vi "test20-LosslessRegisterStateMultipleTimes.vi"(8 "error in (no error)":errorcluster, 11 "TestCase in":refnum<class "testcase-CSMBroadcast.lvclass">) -> (0 "error out":errorcluster, 3 "TestCase out":refnum<class "testcase-CSMBroadcast.lvclass">)   [LabVIEW 2017, in "testcase-CSMBroadcast.lvclass"]
uses:
  testcase-CSMBroadcast.lvclass
  bc269a46-fbd8-4fbd-ac76-06990d02385a.vi
  8d37a2f4-20d8-4102-818c-5a8acec6f80e.vi
  src/user.lib/_NEVSTOP/Communicable State Machine(CSM)/AdvanceAPI/CSM - Get Module Attribute.vi
  <vilib>/addons/_JKI Toolkits/VI Tester/TestCase.llb/TestCase.lvclass
  src/user.lib/_NEVSTOP/Communicable State Machine(CSM)/Communicable State Machine.lvlib
  C:/Program Files (x86)/National Instruments/LabVIEW 2017/vi.lib/addons/_JKI Toolkits/VI Tester/TestCase.llb/TestCase.lvclass
panel:
  out "error out 2":errorcluster
  out "LoopCount":i32
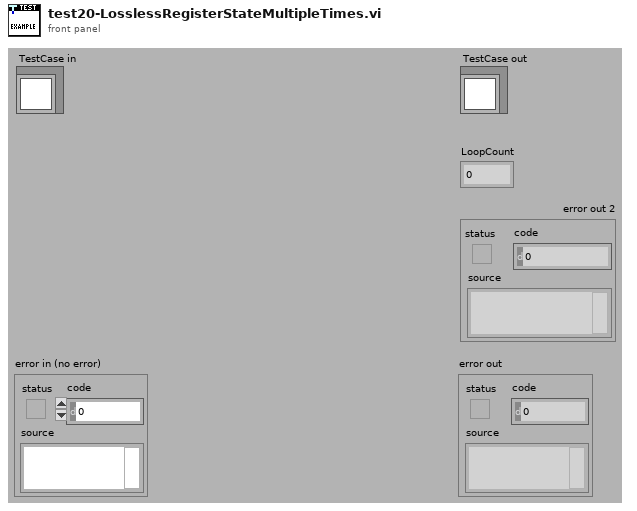
[diagram p1: front panel]
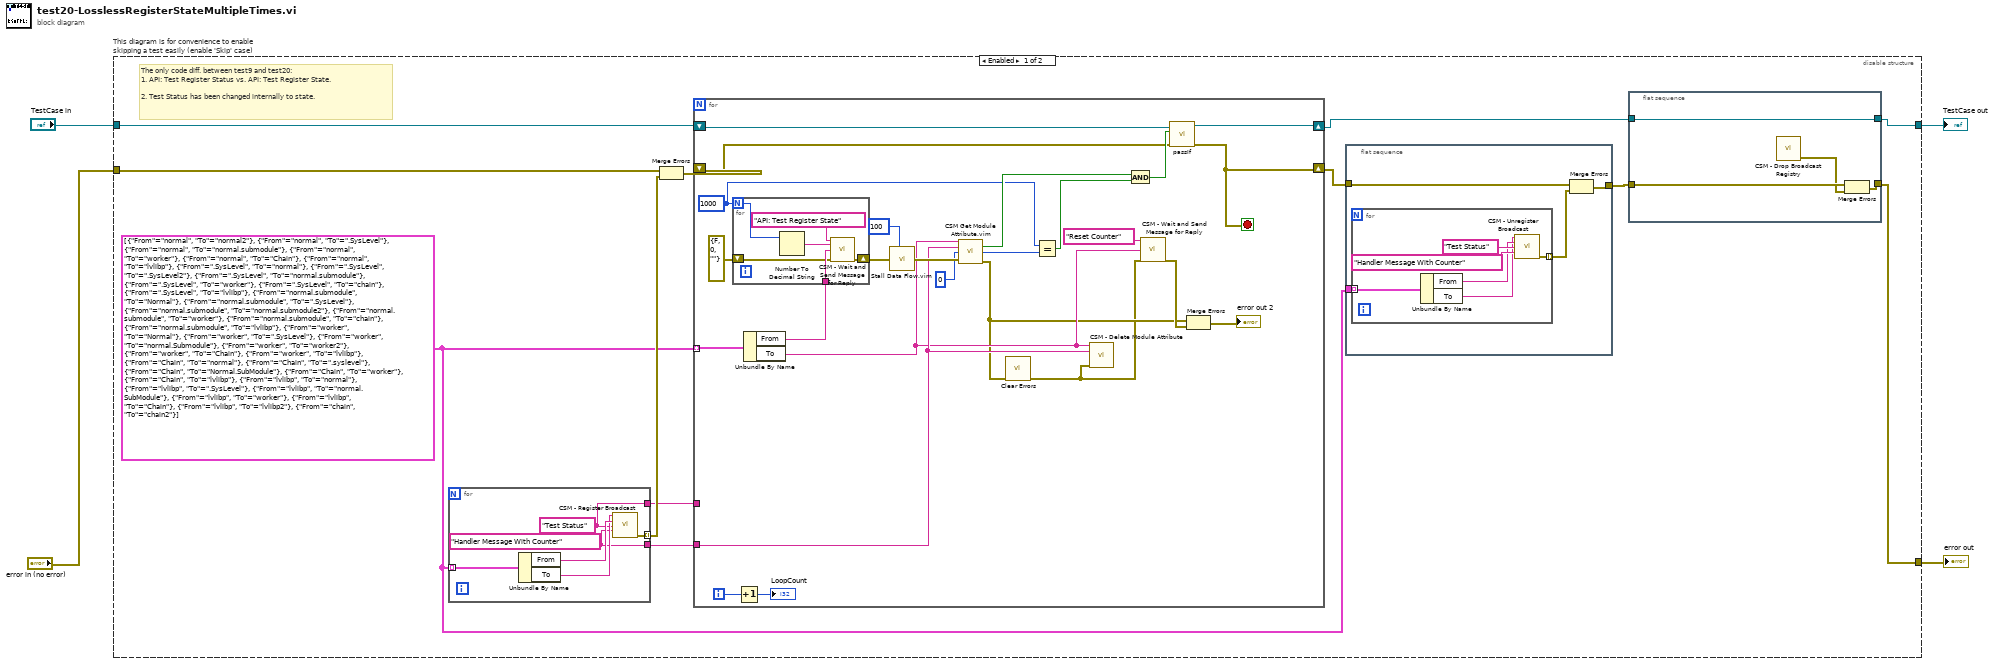
[diagram p0: block diagram]
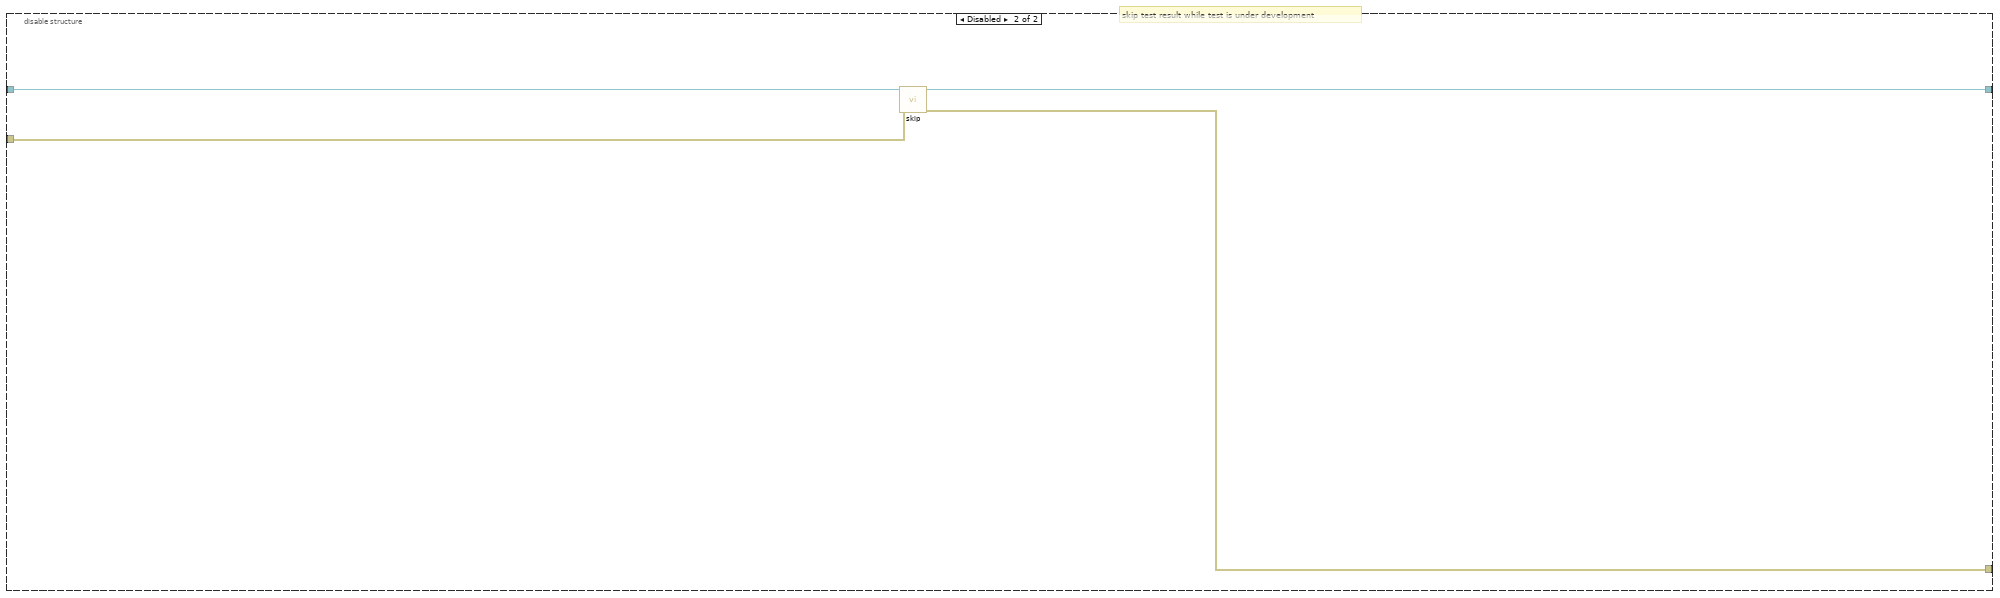
[diagram p2: hidden frame]
diagram:
  n1 = disable-structure "This diagram is for convenience to enable skipping a test easily (enable 'Skip' case)" shown="Enabled" {
    disable-tunnel: "TestCase in" -> [w16 w71]
    disable-tunnel: [w6 w69] -> w2
    disable-tunnel: [w9 w70] -> w1
    disable-tunnel: "error in (no error)" -> [w15 w68]
    frame Enabled {
      w12 = cluster{"From":string, "To":string}[] [{"From"="normal", "To"="normal2"}, {"From"="normal", "To"=".SysLevel"}, {"From"="normal", "To"="normal.submodule"}, {"From"="normal", "To"="worker"}, {"From"="normal", "To"="Chain"}, {"From"="normal", "To"="lvlibp"}, {"From"=".SysLevel", "To"="normal"}, {"From"=".SysLevel", "To"=".SysLevel2"}, {"From"=".SysLevel", "To"="normal.submodule"}, {"From"=".SysLevel", "To"="worker"}, {"From"=".SysLevel", "To"="chain"}, {"From"=".SysLevel", "To"="lvlibp"}, {"From"="normal.submodule", "To"="Normal"}, {"From"="normal.submodule", "To"=".SysLevel"}, {"From"="normal.submodule", "To"="normal.submodule2"}, {"From"="normal.submodule", "To"="worker"}, {"From"="normal.submodule", "To"="chain"}, {"From"="normal.submodule", "To"="lvlibp"}, {"From"="worker", "To"="Normal"}, {"From"="worker", "To"=".SysLevel"}, {"From"="worker", "To"="normal.Submodule"}, {"From"="worker", "To"="worker2"}, {"From"="worker", "To"="Chain"}, {"From"="worker", "To"="lvlibp"}, {"From"="Chain", "To"="normal"}, {"From"="Chain", "To"=".syslevel"}, {"From"="Chain", "To"="Normal.SubModule"}, {"From"="Chain", "To"="worker"}, {"From"="Chain", "To"="lvlibp"}, {"From"="lvlibp", "To"="normal"}, {"From"="lvlibp", "To"=".SysLevel"}, {"From"="lvlibp", "To"="normal.SubModule"}, {"From"="lvlibp", "To"="worker"}, {"From"="lvlibp", "To"="Chain"}, {"From"="lvlibp", "To"="lvlibp2"}, {"From"="chain", "To"="chain2"}]
      # "The only code diff. between test9 and test20:\n1. API: Test Register Status vs. API: Test Register State.\n\n2. Test Status has been changed internally to state."
      n2 = for {
        tunnel: w12 -> [w32] mode=indexing
        tunnel: [w29] -> w13 mode=indexing
        tunnel: [w28] -> w8
        tunnel: [w27] -> w5
        w27 = "Handler Message With Counter" ("Response Message (If \"\", Same as Source Message)")
        w28 = "Test Status" ("Status")
        n3 = Unbundle By Name(w32) -> ("From"=w31:string, "To"=w30:string)
        n4 = call "CSM - Register Broadcast.vi"("CSM Name(Empty for Broadcast Event)"=w30, "Source CSM Name (* as Default)"=w31, "Trigger"=w28, "API (If \"\", Same as Trigger)"=w27) -> ("error out"=w29:errorcluster)  [unwired: 10 in, 1 out]
      }
      n5 = Merge Errors(w15, w13) -> (w14:errorcluster)
      n6 = for {
        tunnel: w12 -> [w61] mode=indexing
        shift-right: [w54] -> w7
        shift-left: w16 -> [w55]
        shift-right: [w51] -> w11
        shift-left: w14 -> [w52]
        tunnel: w8 -> [_]
        tunnel: w5 -> [w50]
        i -> [w49]
        stop <- w51 stop-if-true
        w44 = 1000
        n7 = Increment(x=w49) -> (x+1=→"LoopCount":i32)
        n8 = Unbundle By Name(w61) -> ("From"=w56:string, "To"=w41:string)
        n9 = for {
          N: w44 -> [w62]
          tunnel: w56 -> [w65]
          shift-right: [w66] -> w60
          shift-left: errorcluster {"status"=FALSE, "code"=0, "source"=""} ("error out") -> [w64]
          n10 = Number To Decimal String(number=w62) -> (decimal integer string=w63:string)  [unwired: 1 in]
          n11 = call "CSM - Wait and Send Message for Reply.vi"("State"="API: Test Register State", "Arguments (\"\")"=w63, "Target Module"=w65, "Error In (No Error)"=w64) -> ("error out"=w66:errorcluster)  [unwired: 9 in, 2 out]
        }
        n12 = call "Stall Data Flow.vim"("value in"=w60, "milliseconds to wait"=u32 100) -> ("value out"=w58:errorcluster)  [unwired: 1 out]
        n13 = call "CSM Get Module Attribute.vim"("CSM Name"=w41, "Attribute"=w50, "Default Value (Empty Variant)"=u32 0, "Error In"=w58) -> ("Found"=w57:bool, "Value"=w45:u32, "error out"=w38:errorcluster)  [unwired: 7 in, 2 out]
        n14 = call <vilib>:"Clear Errors.vi"("error in (no error)"=w38) -> ("error out"=w37:errorcluster)  [unwired: 5 in, 1 out]
        n15 = Equal?(x=w44, y=w45) -> (x = y?=w43:bool)
        n16 = call "CSM - Delete Module Attribute.vi"("CSM Name"=w41, "Attribute"=w50, "Error In"=w37) -> ()  [unwired: 9 in, 4 out]
        n17 = Compound Arithmetic op=AND(w57, w43) -> (w53:bool)
        n18 = call "CSM - Wait and Send Message for Reply.vi"("State"="Reset Counter", "Target Module"=w41, "Error In (No Error)"=w37) -> ("error out"=w40:errorcluster)  [unwired: 10 in, 2 out]
        n19 = call-dynamic "passIf.vi"("error in (no error)"=w52, "pass"=w53, "TestCase in"=w55) -> ("error out"=w51:errorcluster, "TestCase out"=w54:refnum<class "testcase-CSMBroadcast.lvclass">)  [unwired: 7 in]
        n20 = Merge Errors(w38, w40) -> (→"error out 2":errorcluster)
      }
      n21 = flat-sequence {
        tunnel: w12 -> [w17]
        tunnel: w11 -> [w20]
        tunnel: [w19] -> w10
        frame #0 {
          n22 = for {
            tunnel: w17 -> [w21] mode=indexing
            tunnel: [w22] -> w18 mode=indexing
            n23 = Unbundle By Name(w21) -> ("From"=w24:string, "To"=w23:string)
            n24 = call "CSM - Unregister Broadcast.vi"("CSM Name(Empty for Broadcast Event)"=w23, "Source CSM Name (* as Default)"=w24, "Trigger"="Test Status" ("Status"), "API (\"*\" as Default)"="Handler Message With Counter" ("Response Message (If \"\", Same as Source Message)")) -> ("error out"=w22:errorcluster)  [unwired: 10 in, 1 out]
          }
          n25 = Merge Errors(w20, w18) -> (w19:errorcluster)
        }
      }
      n26 = flat-sequence {
        tunnel: w10 -> [w36]
        tunnel: [w35] -> w9
        tunnel: [w34] -> w6
        tunnel: w7 -> [w34]
        frame #0 {
          n27 = call "CSM - Drop Broadcast Registry.vi"() -> ("error out"=w33:errorcluster)  [unwired: 15 in]
          n28 = Merge Errors(w36, w33) -> (w35:errorcluster)
        }
      }
    }
    frame Disabled {
      # "skip test result while test is under development"
      n29 = call <vilib>:"skip.vi"("error in (no error)"=w68, "TestCase in"=w71) -> ("error out"=w70:errorcluster, "TestCase out"=w69:refnum<class "testcase-CSMBroadcast.lvclass">)  [unwired: 8 in]
    }
  }
  "error out" <- w1
  "TestCase out" <- w2
